vi "class_data.vi"() -> ()   [LabVIEW 2010, in "GenericStimulator.lvclass"]
uses:
  GenericStimulator.lvclass
panel:
  in  "latest instance":refnum<class "GenericStimulator.lvclass">
  in  "locked by":string
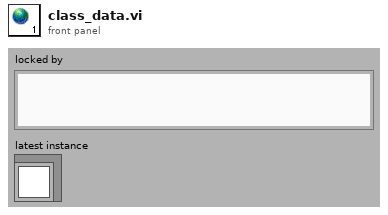
[diagram p1: front panel]
diagram:
